vi "실습 5-2 원그리기.vi"() -> ()   [LabVIEW 2014]
uses:
  <vilib>/Analysis/NI_AALBase.lvlib
panel:
  out "XY 그래프":cluster{"sine wave":dbl[], "sine wave":dbl[]}[](graph)
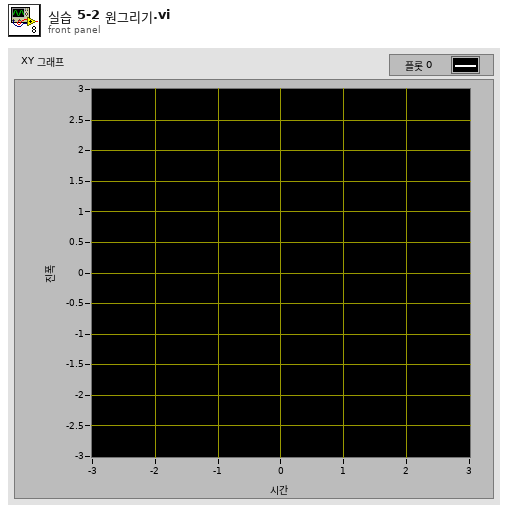
[diagram p1: front panel]
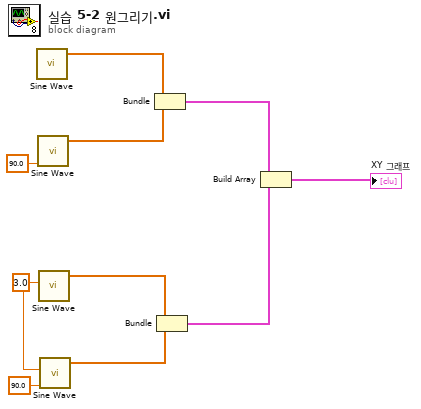
[diagram p0: block diagram]
diagram:
  w4 = 3.0 ("amplitude")
  n1 = call <vilib>:"Sine Wave.vi"() -> ("sine wave"=w9:dbl[])  [unwired: 5 in, 2 out]
  n2 = call <vilib>:"Sine Wave.vi"("phase in"=90.0) -> ("sine wave"=w8:dbl[])  [unwired: 4 in, 2 out]
  n3 = call <vilib>:"Sine Wave.vi"("amplitude"=w4) -> ("sine wave"=w6:dbl[])  [unwired: 4 in, 2 out]
  n4 = call <vilib>:"Sine Wave.vi"("amplitude"=w4, "phase in"=90.0) -> ("sine wave"=w7:dbl[])  [unwired: 3 in, 2 out]
  n5 = Bundle("sine wave"=w9, "sine wave"=w8) -> (w3:cluster{"sine wave":dbl[], "sine wave":dbl[]})  [unwired: 1 in]
  n6 = Bundle("sine wave"=w6, "sine wave"=w7) -> (w2:cluster{"sine wave":dbl[], "sine wave":dbl[]})  [unwired: 1 in]
  n7 = Build Array(w3, w2) -> (→"XY 그래프":cluster{"sine wave":dbl[], "sine wave":dbl[]}[])
